vi "Global CAMBIO CTRL FRENO.vi"() -> ()   [LabVIEW 2019]
panel:
  out "CAMBIO CTRL IN CORSO":bool
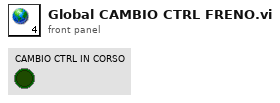
[diagram p1: front panel]
diagram:
